vi "comm status flags.vi"(1 "Status Flags":u32 format="%.0x") -> (0 "status flags cluster":T1)   [LabVIEW 2013, in "lvserial.lvlib"]
doc: "Decodes the error flags from Comm Status.vi"
uses:
  lvserial.lvlib
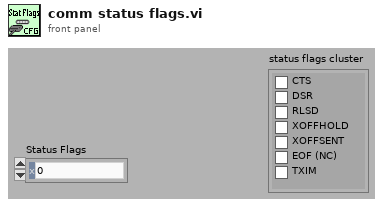
[diagram p1: front panel]
types:
  T1 = cluster{"CTS":bool, "DSR":bool, "RLSD":bool, "XOFFHOLD":bool, "XOFFSENT":bool, "EOF (NC)":bool, "TXIM":bool}
  T2 = cluster{"Boolean array[0]":bool, "Boolean array[1]":bool, "Boolean array[2]":bool, "Boolean array[3]":bool, "Boolean array[4]":bool, "Boolean array[5]":bool, "Boolean array[6]":bool}
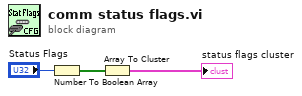
[diagram p0: block diagram]
diagram:
  n1 = Number To Boolean Array(number="Status Flags") -> (Boolean array=w2:bool[])
  n2 = Array To Cluster(array=w2) -> (cluster=→"status flags cluster":T2)
